vi "LED Lighting Effect.vi"(5 "Interval (mS)":u32, 7 "Duration (mS, Default: Inf)":u32, 8 "error in (no error)":errorcluster, 10 "Lighting Effect":T1, 11 "LED Color":u32(colorbox)) -> (0 "error out":errorcluster)   [LabVIEW 2022 SP3, in "Logitech Devices.lvlib"]
uses:
  Logitech Devices.lvlib
  C:/Program Files/LGHUB/sdks/sdk_legacy_led_x86.dll
  TypeDefs/Lighting Effects.ctl
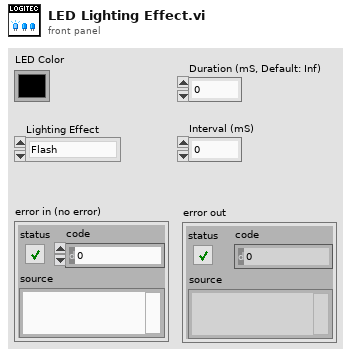
[diagram p1: front panel]
types:
  T1 = typedef "Logitech Devices.lvlib/Lighting Effects.ctl" = enum8{"Flash", "Pulse"}
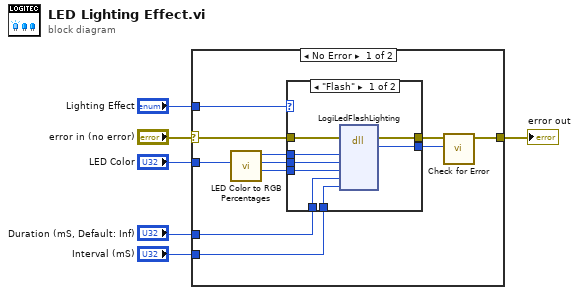
[diagram p0: block diagram]
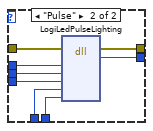
[diagram p2: hidden frame]
diagram:
  n1 = case shown="No Error" "error in (no error)" {
    selector: "error in (no error)" -> [w17 w34]
    tunnel: [w7 w34] -> w5
    tunnel: "LED Color" -> [w15 _]
    tunnel: "Lighting Effect" -> [w14 _]
    tunnel: "Duration (mS, Default: Inf)" -> [w10 _]
    tunnel: "Interval (mS)" -> [w9 _]
    frame No Error {
      n2 = call "LED Color to RGB Percentages.vi"("LED Color"=w15) -> ("Blue %"=w11:u8, "Green %"=w12:u8, "Red %"=w13:u8)  [unwired: 8 in]
      n3 = case shown="\"Flash\"" w14 {
        tunnel: w17 -> [w25 w33]
        tunnel: [w24 w32] -> w8
        tunnel: [w23 w31] -> w16
        tunnel: w13 -> [w22 w30]
        tunnel: w12 -> [w21 w29]
        tunnel: w11 -> [w20 w28]
        tunnel: w10 -> [w19 w27]
        tunnel: w9 -> [w18 w26]
        frame "Flash" {
          n4 = dll-call lib="C:/Program Files/LGHUB/sdks/sdk_legacy_led_x86.dll" fn="LogiLedFlashLighting"(error in=w25, "Red Percentage"=w22, "Green Percentage"=w21, "Blue Percentage"=w20, "Duration"=w19, "Interval"=w18) -> (error out=w24:errorcluster, "return type"=w23:u8)  [unwired: 7 in, 1 out]
        }
        frame "Pulse" {
          n5 = dll-call lib="C:/Program Files/LGHUB/sdks/sdk_legacy_led_x86.dll" fn="LogiLedPulseLighting"(error in=w33, "Red Percentage"=w30, "Green Percentage"=w29, "Blue Percentage"=w28, "Duration"=w27, "Interval"=w26) -> (error out=w32:errorcluster, "return type"=w31:u8)  [unwired: 7 in, 1 out]
        }
      }
      n6 = call "Check for Error.vi"("DLL-call return value"=w16, "error in (no error)"=w8) -> ("error out"=w7:errorcluster)  [unwired: 9 in]
    }
    frame Error {
    }
  }
  "error out" <- w5
